vi "GetRefrigPressures.vi"(8 "error in":errorcluster, 10 "Refrig system number (1-4)":T1=1 items=["Channel 1"=1, "Channel 2"=2, "Channel 3"=3, "Channel 4"=4], 11 "VISA resource name":refnum<visa-resource-name>) -> (0 "error out":errorcluster, 2 "Refrig system pressures":string, 3 "VISA resource name out":refnum<visa-resource-name>)   [LabVIEW 2023, in "Thermotron 8800.lvlib"]
doc: "REFG\nCommand name: Send refrigeration system pressures\nCommand type: System status\nDescription: When used, “n” is the refrigeration system number (1, 2, 3, or 4). When “n” is not used, the 8800 defaults to system 1. The 8800 returns four pressures and four temperatures in integer format, and a binary-coded decimal refrigeration mode word. The pressures are in psi and the temperatures are in Celsius. The string breaks down as follows:\n• Four pressures for high-stage suction, high-stage discharge, low-stage suction, and low-stage discharge.\n• Four temperatures for high-stage suction, high-stage discharge, low-stage suction, and low-stage discharge.\n• One coded integer that indicates the refrigeration mode. Each mode has its own weighting value:\n1 Humidity cooling mode \n2 Temperature cooling mode \n4 Cascade mode \n8 Pump-down mode \n16 High-stage compressor trip \n32 Low-stage compressor trip\nFor example, a 6 (4 + 2) indicates the 8800 is in cascade and temperature cooling modes.\nSyntax: REFG(n)?\nData type: String (NOTE: The first four variables in the string are integers, the next four variables are one-decimal-place real numbers, and the final variable is an integer.)\nQuery example: REFG?\n8800 response: 25,220,25,249,-23.2,87.5,-23.6,113.4,6. This string indicates the following:\n• High-stage suction pressure 25, high-stage discharge pressure 220, low-stage suction pressure 25, and low-stage discharge pressure 249.\n• High-stage suction temperature -23.2, high-stage discharge temperature 87.5, low-stage suction temperature -23.6, and low-stage discharge temperature 113.4.\n• Refrigeration mode: cascade and temperature cooling."
uses:
  Thermotron 8800.lvlib
  Private/AnalogInputChannelNumber 1-4.ctl
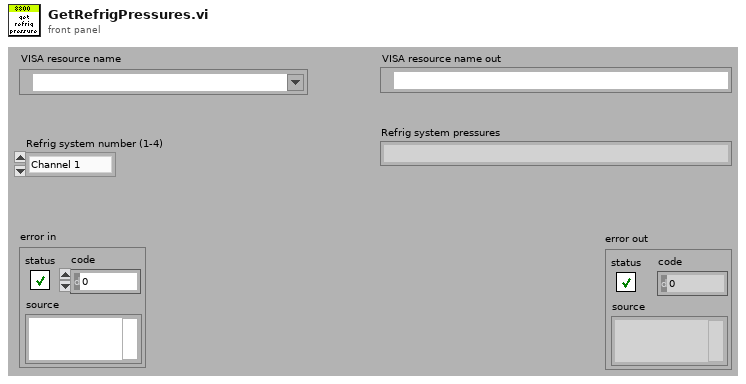
[diagram p1: front panel]
types:
  T1 = typedef "Thermotron 8800.lvlib/AnalogInputChannelNumber 1-4.ctl" = u16
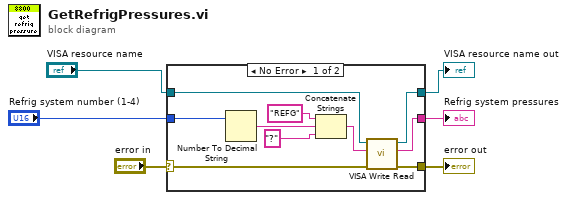
[diagram p0: block diagram]
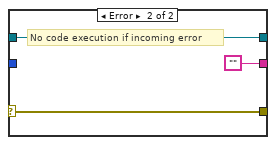
[diagram p2: hidden frame]
diagram:
  n1 = case shown="No Error" "error in" {
    selector: "error in" -> [w12 w19]
    tunnel: [w11 w19] -> w5
    tunnel: "Refrig system number (1-4)" -> [w10 _]
    tunnel: "VISA resource name" -> [w9 w17]
    tunnel: [w8 w17] -> w3
    tunnel: [w7 ""] -> w2
    frame No Error {
      n2 = Number To Decimal String(number=w10) -> (decimal integer string=w16:string)  [unwired: 1 in]
      n3 = Concatenate Strings("REFG" ("8800 Command"), w16, "?" ("8800 Command")) -> (w15:string)
      n4 = call "VISA Write Read.vi"("error in (no error)"=w12, "8800 Command"=w15, "VISA Refnum in"=w9) -> ("error out"=w11:errorcluster, "read buffer"=w7:string, "VISA Refnum out"=w8:refnum<visa-resource-name>)  [unwired: 6 in]
    }
    frame Error {
      # "No code execution if incoming error"
    }
  }
  "error out" <- w5
  "VISA resource name out" <- w3
  "Refrig system pressures" <- w2
